vi "FTW-JSON-Object-DeleteElement.vi"(0 "JSON Object":refnum<class "FTW-JSON.lvclass">, 5 "Key":string, 11 "error in":errorcluster) -> (4 "JSON Object out":refnum<class "FTW-JSON.lvclass">, 6 "Found?":bool, 15 "error out":errorcluster)   [LabVIEW 2012, in "FTW-JSON.lvclass"]
uses:
  FTW-JSON.lvclass
  FTW-JSON.lvclass/FTW-JSON.ctl
panel:
  # "Inputs"
  # "Outputs"
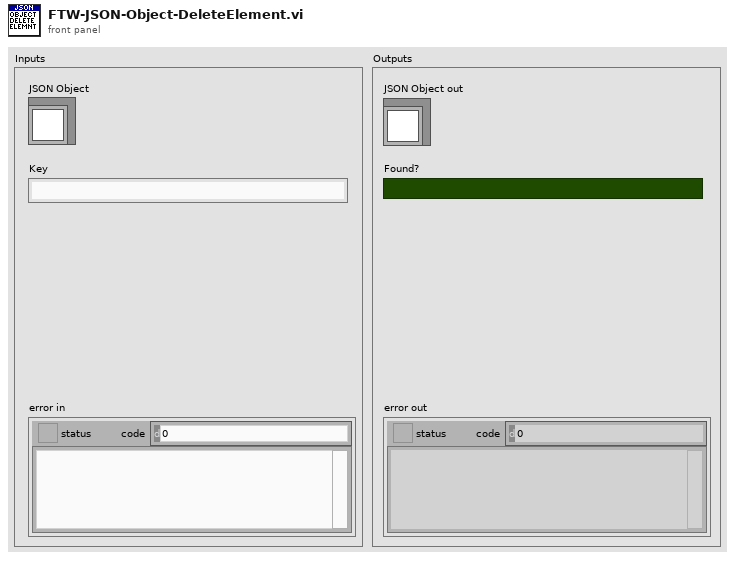
[diagram p1: front panel]
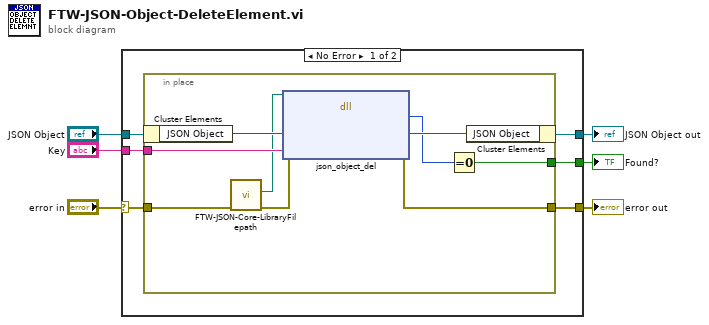
[diagram p0: block diagram]
diagram:
  n1 = case shown="No Error" "error in" {
    selector: "error in" -> [w12 w23]
    tunnel: [w8 w23] -> w6
    tunnel: [w10 w22] -> w4
    tunnel: "JSON Object" -> [w11 w22]
    tunnel: "Key" -> [w9 _]
    tunnel: [w7 _] -> w1
    frame No Error {
      n2 = in-place {
        in-place-border: w12 -> [w21]
        in-place-border: w9 -> [w19]
        in-place-border: [w16] -> w8
        in-place-border: [w13] -> w7
        n3 = in-place-cluster #1(w11) -> ("JSON Object"=w20:i64)
        n4 = call "FTW-JSON-Core-LibraryFilepath.vi"("error in"=w21) -> ("error out"=w18:errorcluster, "JSON Library Filepath"=w17:path)  [unwired: 9 in]
        n5 = dll-call lib="?" fn="json_object_del"(path in=w17, error in=w18, "JSON Object Pointer"=w20, "Element Key"=w19) -> (error out=w16:errorcluster, "JSON Element Pointer"=w14:i64, "JSON Object Pointer"=w15:i64)  [unwired: 2 in, 1 out]
        n6 = Equal To 0?(x=w14) -> (x = 0?=w13:bool)
        n7 = in-place-cluster #1("JSON Object"=w15) -> (w10:refnum<class "FTW-JSON.lvclass">)
      }
    }
    frame Error {
    }
  }
  "error out" <- w6
  "JSON Object out" <- w4
  "Found?" <- w1
